vi "Configure Action Core.vi"(8 "error in (no error)":errorcluster, 11 "NI DAQmx AI Voltage in":refnum<class "NI DAQmx AI Voltage.lvclass">) -> (0 "error out":errorcluster, 3 "NI DAQmx AI Voltage out":refnum<class "NI DAQmx AI Voltage.lvclass">)   [LabVIEW 2023, in "NI DAQmx AI Voltage.lvlib" / "NI DAQmx AI Voltage.lvclass"]
uses:
  NI DAQmx AI Voltage.lvclass
  NI DAQmx AI Voltage.lvclass/NI DAQmx AI Voltage.ctl
  <vilib>/DAQmx/create/channels.llb/DAQmx Create Channel (AI-Voltage-Basic).vi
  <vilib>/DAQmx/configure/timing.llb/DAQmx Timing (Sample Clock).vi
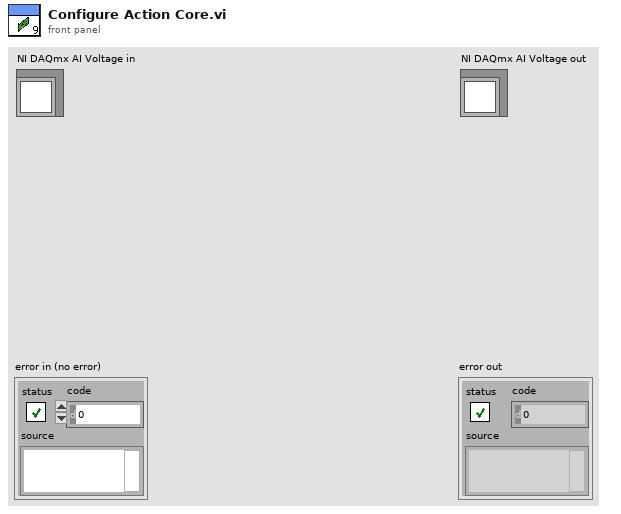
[diagram p1: front panel]
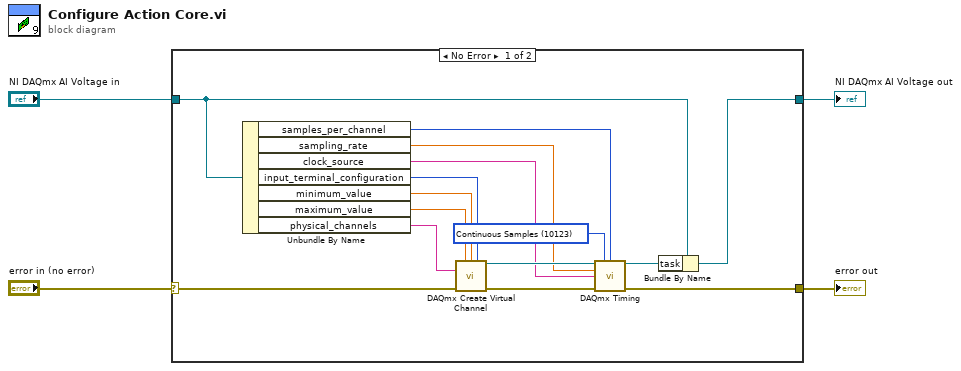
[diagram p0: block diagram]
diagram:
  n1 = case shown="No Error" "error in (no error)" {
    selector: "error in (no error)" -> [w19 w21]
    tunnel: [w8 w21] -> w3
    tunnel: "NI DAQmx AI Voltage in" -> [w7 w20]
    tunnel: [w5 w20] -> w1
    frame No Error {
      w10 = 10123 items=["Finite Samples"=10178, "Continuous Samples"=10123, "Hardware Timed Single Point"=12522] ("sample mode")
      n2 = Unbundle By Name(w7) -> ("samples_per_channel"=w9:i32, "sampling_rate"=w11:dbl, "clock_source"=w12:string, "input_terminal_configuration"=w18:i32, "minimum_value"=w17:dbl, "maximum_value"=w16:dbl, "physical_channels"=w15:string)
      n3 = call-poly <vilib>:"DAQmx Create Virtual Channel.vi"("maximum value"=w16, "minimum value"=w17, "input terminal configuration"=w18, "physical channels"=w15, "error in"=w19) -> ("task out"=w13:refnum<k21>, "error out"=w14:errorcluster)  [unwired: 9 in]
      n4 = call-poly <vilib>:"DAQmx Timing.vi"("task/channels in"=w13, "sample mode"=w10, "samples per channel"=w9, "rate"=w11, "source"=w12, "error in"=w14) -> ("task out"=w6:refnum<k21>, "error out"=w8:errorcluster)  [unwired: 8 in]
      n5 = Bundle By Name(cluster=w7, "task"=w6) -> (w5:refnum<class "NI DAQmx AI Voltage.lvclass">)
    }
    frame Error {
    }
  }
  "error out" <- w3
  "NI DAQmx AI Voltage out" <- w1
